vi "ExConvertFile.vi"() -> ()   [LabVIEW 2010]
panel:
  in  "Output File Operation":u32=9
  in  "Output File Name":string
  in  "Output FileType":u32=67174400
  in  "stop":bool
  in  "Input File Operation":u32=6
  in  "Input File Name":string
  in  "Input FileType":u32=67371008
  out "error out":errorcluster
  in  "error in (no error)":errorcluster
  # "TIF   = 67174400\n  SPE = 67371008\n  PMI  = 67436544"
  # "6 = Read Only"
  # "TIF   = 67174400\n  SPE = 67371008\n  PMI  = 67436544"
  # "9 = Open New / Write Only"
  # "ExConvertFile.vi\nThis VI will open the input file, display it and save\nit to the output file.  Note that the full path names\nmust be provided for both input and output files.\n\nThe STOP button must be used to end this VI.\nIt will correctly close the display window."
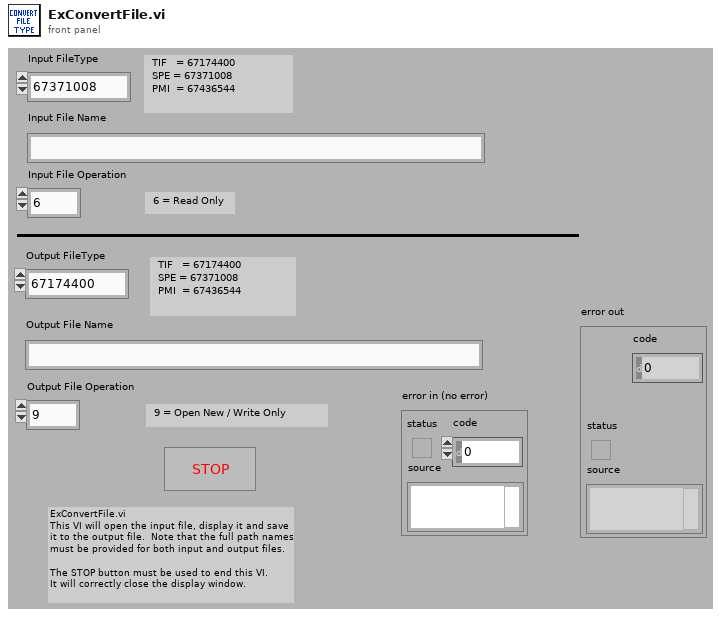
[diagram p1: front panel]
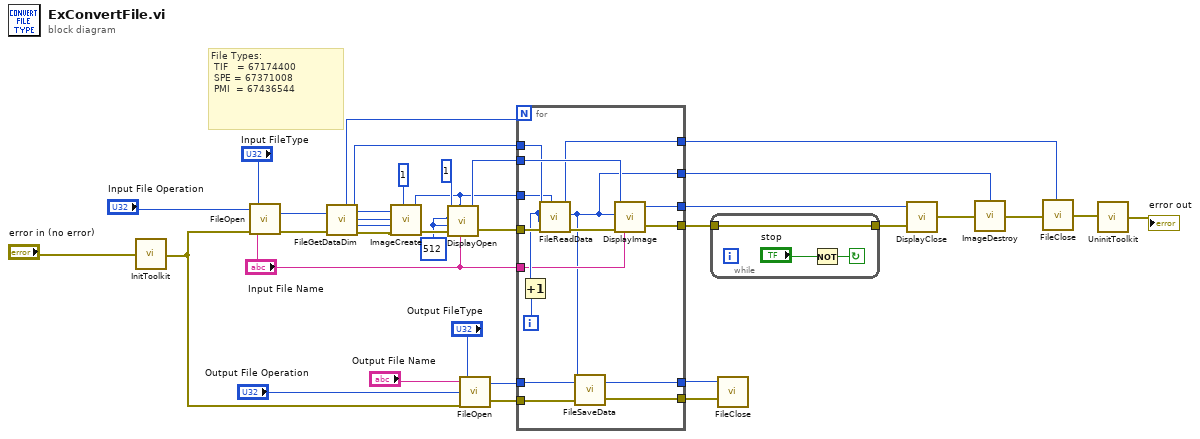
[diagram p0: block diagram]
diagram:
  w25 = 512
  # "File Types:\n TIF   = 67174400\n SPE = 67371008\n PMI  = 67436544"
  n1 = call <userlib>:"InitToolkit.vi"("error in"="error in (no error)") -> ("error out"=w7:errorcluster)
  n2 = call <userlib>:"FileOpen.vi"("error in"=w7, "File Operations"="Input File Operation", "FileName"="Input File Name", "File Type"="Input FileType") -> ("error out"=w34:errorcluster, "File Handle"=w33:u32)
  n3 = call <userlib>:"FileGetDataDim.vi"("File Handle"=w33, "error in"=w34) -> ("Number of Frames"=w27:u32, "Data Type"=w29:u32, "File Handle"=w21:u32, "X dim"=w31:u32, "Y dim"=w30:u32, "error out"=w32:errorcluster)
  n4 = call <userlib>:"ImageCreate.vi"("X dimension"=w31, "Y dimension"=w30, "Data Type"=w29, "error in"=w32, "Number Of Frames"=1) -> ("Image Handle"=w20:u32, "error out"=w28:errorcluster)
  n5 = call <userlib>:"DisplayOpen.vi"("Display Title"="Input File Name", "Image Handle"=w20, "error in"=w28, "Display Height"=w25, "Display Width"=w25, "Display Type"=1) -> ("error out"=w23:errorcluster, "Display Handle"=w22:u32)
  n6 = call <userlib>:"FileOpen.vi"("error in"=w7, "File Operations"="Output File Operation", "FileName"="Output File Name", "File Type"="Output FileType") -> ("error out"=w5:errorcluster, "File Handle"=w6:u32)
  n7 = for {
    N: w27 -> [_]
    tunnel: w23 -> [w52]
    tunnel: w22 -> [w50]
    tunnel: w21 -> [w49]
    tunnel: w20 -> [w48]
    tunnel: [w42] -> w12
    tunnel: [w45] -> w19
    tunnel: [w44] -> w18
    tunnel: [w41] -> w15
    tunnel: "Input File Name" -> [w43]
    tunnel: w6 -> [w40]
    tunnel: [w39] -> w4
    tunnel: w5 -> [w38]
    tunnel: [w37] -> w3
    i -> [w47]
    n8 = Increment(x=w47) -> (x+1=w46:i32)
    n9 = call <userlib>:"FileReadData.vi"("File Handle"=w49, "Start Frame"=w46, "End Frame"=w46, "error in"=w52, "Image Handle"=w48) -> ("File Handle"=w44:u32, "Image Handle"=w41:u32, "error out"=w51:errorcluster)
    n10 = call <userlib>:"FileSaveData.vi"("error in"=w38, "Image Handle"=w41, "File Handle"=w40) -> ("error out"=w37:errorcluster, "File Handle"=w39:u32)
    n11 = call <userlib>:"DisplayImage.vi"("error in"=w51, "Title"=w43, "Image Handle"=w41, "Display Handle"=w50) -> ("error out"=w42:errorcluster, "Display Handle"=w45:u32)
  }
  n12 = while {
    tunnel: w12 -> [w55]
    tunnel: [w55] -> w13
    stop <- w53 continue-if-true
    n13 = Not(x="stop") -> (.not. x?=w53:bool)
  }
  n14 = call <userlib>:"FileClose.vi"("error in"=w3, "File Handle"=w4) -> ()  [unwired: 1 out]
  n15 = call <userlib>:"DisplayClose.vi"("error in"=w13, "Display Handle"=w19) -> ("error out"=w17:errorcluster)
  n16 = call <userlib>:"ImageDestroy.vi"("error in"=w17, "Data handle"=w15) -> ("error out"=w16:errorcluster)
  n17 = call <userlib>:"FileClose.vi"("error in"=w16, "File Handle"=w18) -> ("error out"=w2:errorcluster)
  n18 = call <userlib>:"UninitToolkit.vi"("error in"=w2) -> ("error out"=→"error out":errorcluster)
